vi "construct_error_object.vi"(7 "error_time (now)":timestamp, 8 "error_to_process":errorcluster, 9 "error_mark":string, 10 "error_type":T1, 11 "error_source":refnum<class>) -> (1 "fire_warning":bool, 2 "fire_error":bool, 3 "Error":refnum<class "Error.lvclass">)   [LabVIEW 2023, in "Error Handling Interface.lvlib" / "Error.lvclass"]
doc: "Use this method to encapsulate information about the error for the error handling module.\nThis will return an Error type object to be transfered to the Error handling application if error_to_process.status == True.\nOtherwise, if error_to_process.code != 0 and error_to_process.status == False, sets output fire_warning = True."
uses:
  Error.lvclass
  error_type.ctl
  Error.lvclass/Error.ctl
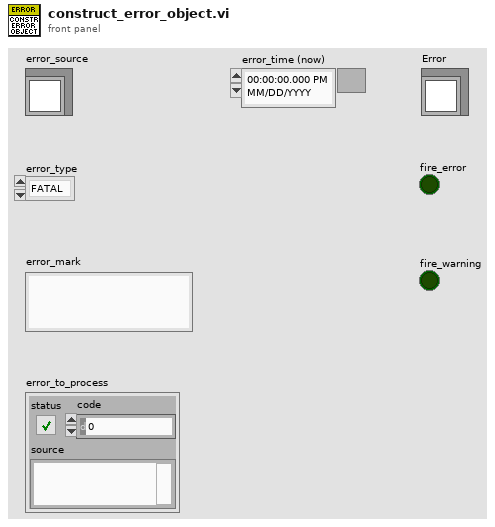
[diagram p1: front panel]
types:
  T1 = typedef "Error Handling Interface.lvlib/Error.lvclass/error_type.ctl" = enum16{"FATAL", "ERROR", "WARNING", "INFO", "DEBUG", "TRACE"}
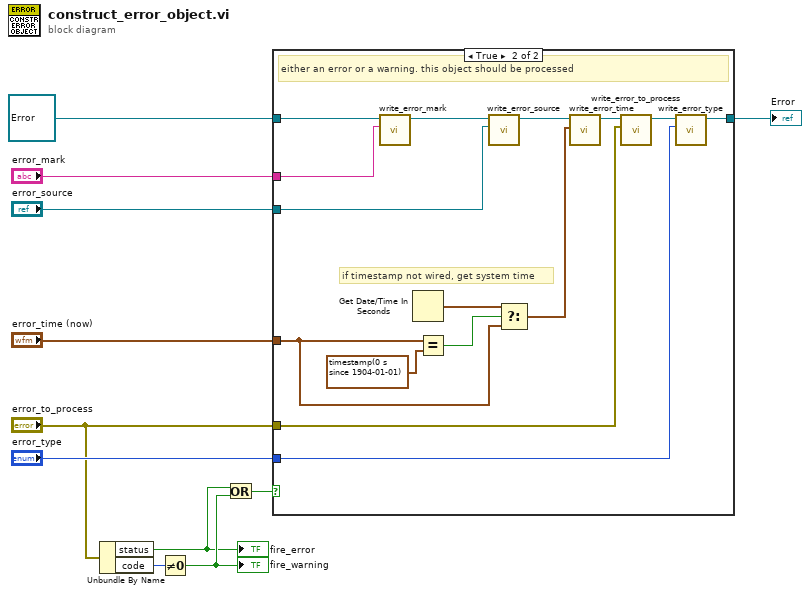
[diagram p0: block diagram]
diagram:
  n1 = Unbundle By Name("error_to_process") -> ("status"=w2:bool, "code"=w4:i32)
  "fire_error" <- w2
  n2 = Not Equal To 0?(x=w4) -> (x != 0?=w3:bool)
  "fire_warning" <- w3
  n3 = Or(x=w2, y=w3) -> (x .or. y?=w1:bool)
  n4 = case shown="True" w1 {
    tunnel: refnum<class "Error.lvclass"> refnum ("Error in") -> [w12 w27]
    tunnel: "error_type" -> [_ w26]
    tunnel: "error_source" -> [_ w25]
    tunnel: "error_mark" -> [_ w24]
    tunnel: [w12 w23] -> w7
    tunnel: "error_time (now)" -> [_ w22]
    tunnel: "error_to_process" -> [_ w21]
    frame False {
      # "This object should not be processed"
    }
    frame True {
      # "if timestamp not wired, get system time"
      # "either an error or a warning. this object should be processed"
      n5 = call "write_error_mark.vi"("error_mark"=w24, "Error in"=w27) -> ("Error out"=w20:refnum<class "Error.lvclass">)  [unwired: 9 in]
      n6 = Get Date/Time In Seconds() -> (seconds since 1Jan1904=w13:timestamp)
      n7 = Equal?(x=w22, y=timestamp(0 s since 1904-01-01)) -> (x = y?=w14:bool)
      n8 = call "write_error_source.vi"("error_source"=w25, "Error in"=w20) -> ("Error out"=w19:refnum<class "Error.lvclass">)  [unwired: 9 in]
      n9 = Select(t=w13, s=w14, f=w22) -> (s? t:f=w15:timestamp)
      n10 = call "write_error_time.vi"("error_time"=w15, "Error in"=w19) -> ("Error out"=w18:refnum<class "Error.lvclass">)  [unwired: 9 in]
      n11 = call "write_error_to_process.vi"("error_to_process"=w21, "Error in"=w18) -> ("Error out"=w17:refnum<class "Error.lvclass">)  [unwired: 9 in]
      n12 = call "write_error_type.vi"("error_type"=w26, "Error in"=w17) -> ("Error out"=w23:refnum<class "Error.lvclass">)  [unwired: 9 in]
    }
  }
  "Error" <- w7
